vi "GetSelectionList.vi"(8 "error in (no error)":errorcluster caption="错误输入（无错误）", 11 "DigitalDisplay 输入":refnum<class "DigitalDisplay.lvclass">) -> (0 "error out":errorcluster caption="错误输出", 3 "DigitalDisplay 输出":refnum<class "DigitalDisplay.lvclass">)   [LabVIEW 2018, in "DataDisplay.lvlib" / "DigitalDisplay.lvclass"]
uses:
  DigitalDisplay.lvclass
  DigitalDisplay.lvclass/DigitalDisplay.ctl
  DataDisplay.lvlib
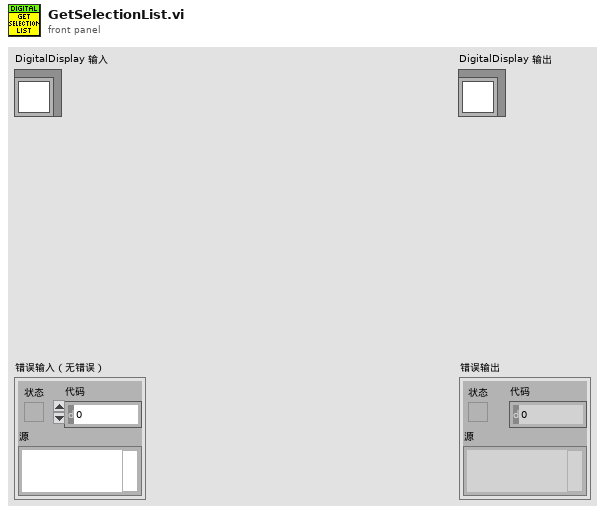
[diagram p1: front panel]
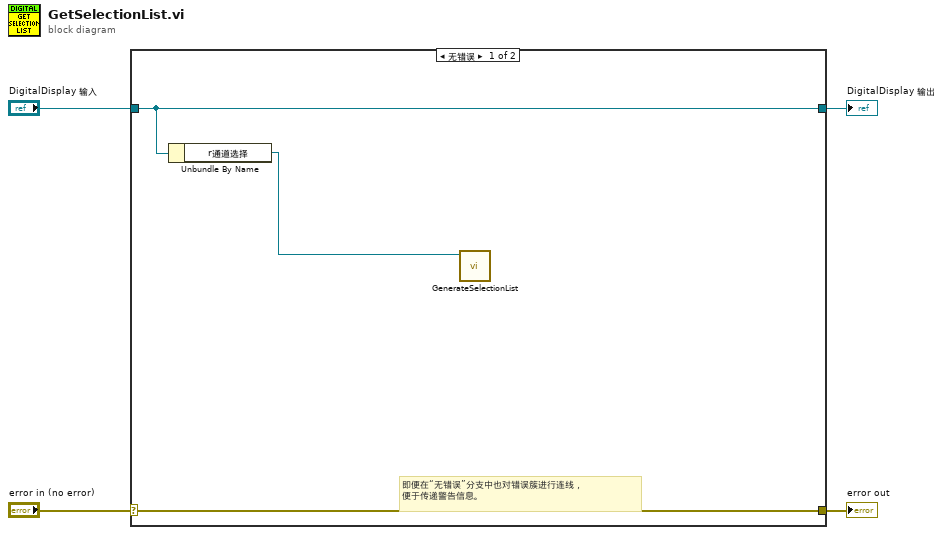
[diagram p0: block diagram]
diagram:
  n1 = case shown="无错误" "error in (no error)" {
    selector: "error in (no error)" -> [w7 w9]
    tunnel: [w7 w9] -> w3
    tunnel: [w6 w8] -> w1
    tunnel: "DigitalDisplay 输入" -> [w6 w8]
    frame No Error {
      # "即便在“无错误”分支中也对错误簇进行连线，\n便于传递警告信息。"
      n2 = Unbundle By Name(w6) -> ("r通道选择"=w5:refnum<vi>)
      n3 = call "GenerateSelectionList.vi"("ref通道选择"=w5) -> ()  [unwired: 11 in]
    }
    frame Error {
    }
  }
  "error out" <- w3
  "DigitalDisplay 输出" <- w1
